vi "EVE.vi"() -> ()   [LabVIEW 2011]
uses:
  <vilib>/express/express analysis/Spectral/XNode/ExpressSpectralMeasurementsBlockNode.xnode
  <vilib>/express/express analysis/Spectral/Block/exnSpectralBlock spectral measurements RMS poly.vi
  <vilib>/picture/3D Picture Control/NI_3D Picture Control.lvlib
  <vilib>/Analysis/NI_AALPro.lvlib
  <vilib>/Analysis/2dsp.llb/Real FFT.vi
  <vilib>/Utility/file.llb/Read From Spreadsheet File (string).vi
  <vilib>/Platform/NI_3dgraph.lvlib
  <vilib>/Analysis/coordinate.llb/3D Cartesian Coordinate Rotation (Euler) (Array).vi
  <vilib>/express/express analysis/Spectral/Block/exnSpectralBlock spectral measurements RMS DDT.vi
  <vilib>/Analysis/4window.llb/Hamming Window (DBL).vi
  <vilib>/imath/engines/lvmath/Plug In/_Char/NIMS_CH_String CV to Character 2D.vi
  <vilib>/imath/engines/lvmath/Plug In/_Char/NIMS_CH_Character 2D to U8 2D.vi
  <vilib>/imath/engines/lvmath2/RunTimeEngine/ArithmeticOperatorToken/NIMS_ArithmeticOperator_multmx.vi
  <vilib>/imath/engines/lvmath2/RunTimeEngine/ArithmeticOperatorToken/NIMS_ArithmeticOperator_plus.vi
  <vilib>/imath/engines/lvmath2/RunTimeEngine/ArithmeticOperatorToken/NIMS_ArithmeticOperator_powermx(M,M).vi
  <vilib>/imathl/engines/lvmath/Functions/Error Handling/Create Error.vi
  <vilib>/imath/engines/lvmath2/RunTimeEngine/BuiltInFunctions/atan2/NIMS_atan2(A,A).vi
  <vilib>/imath/engines/lvmath2/RunTimeEngine/ErrorHandling/NIMS_Create Error From Enums.vi
  <vilib>/imath/engines/lvmath/Functions/Error Handling/MergeErrorsWrapper.vi
  <vilib>/imath/engines/lvmath2/RunTimeEngine/ArithmeticOperatorToken/NIMS_ArithmeticOperator_minus.vi
  <vilib>/imath/engines/lvmath2/RunTimeEngine/NodeEndStatement/NIMS_NodeEndStatement_Output.vi
  <vilib>/imath/engines/lvmath2/RunTimeEngine/ErrorHandling/NIMS_Finalize Error.vi
panel:
  out "Z direction  FFT 10":dbl[](graph)
  out "Z direction  FFT 9":dbl[](graph)
  out "Z direction  FFT 8":dbl[](graph)
  out "Z direction  FFT 7":dbl[](graph)
  out "Z direction  FFT 6":dbl[](graph)
  out "Z direction  FFT 5":dbl[](graph)
  in  "3D Curve":refnum<k7>(container)
  in  "Z":dbl[](array[numeric])
  in  "Y":dbl[](array[numeric])
  in  "X":dbl[](array[numeric])
  out "Z direction  FFT 4":dbl[](graph)
  out "Y direction  FFT":dbl[](graph)
  out "X direction  FFT 2":dbl[](graph)
  out "Data Selected 3":u16
  out "Data Selected 2":u16
  in  "Load in CSV File Data1":path
  in  "Tab Control 2":enum32{"Swimming", "Cycling", "Running"}(tab)
  in  "Tab Control":enum32{"Raw Accelerations", "FFT"}(tab)
  in  "Select Data to Analyse":u16(ring) items=["Data 0", "Data 1"]
  in  "Angle":sgl(knob) scale=0.0..360.0
  in  "Axis":cluster{"X":sgl, "Y":sgl, "Z":sgl}
  out "?":string[](array[string])
  out "?":string[](array[string])
  out "Data Seperated and Organised into Columns and Rows":string[][](array[string])
  out "CSV File":string[][](array[string])
  in  "Stop":bool
  out "Number of Rows in File":i32
  in  "Load in CSV File Data0":path
  in  "Translation":cluster{"X":sgl, "Y":sgl, "Z":sgl}
  out "3D Picture Control":refnum<vi>(3d-picture)
  in  "stop":bool
  in  "STL File Path":path
  in  "Reset Signal":bool
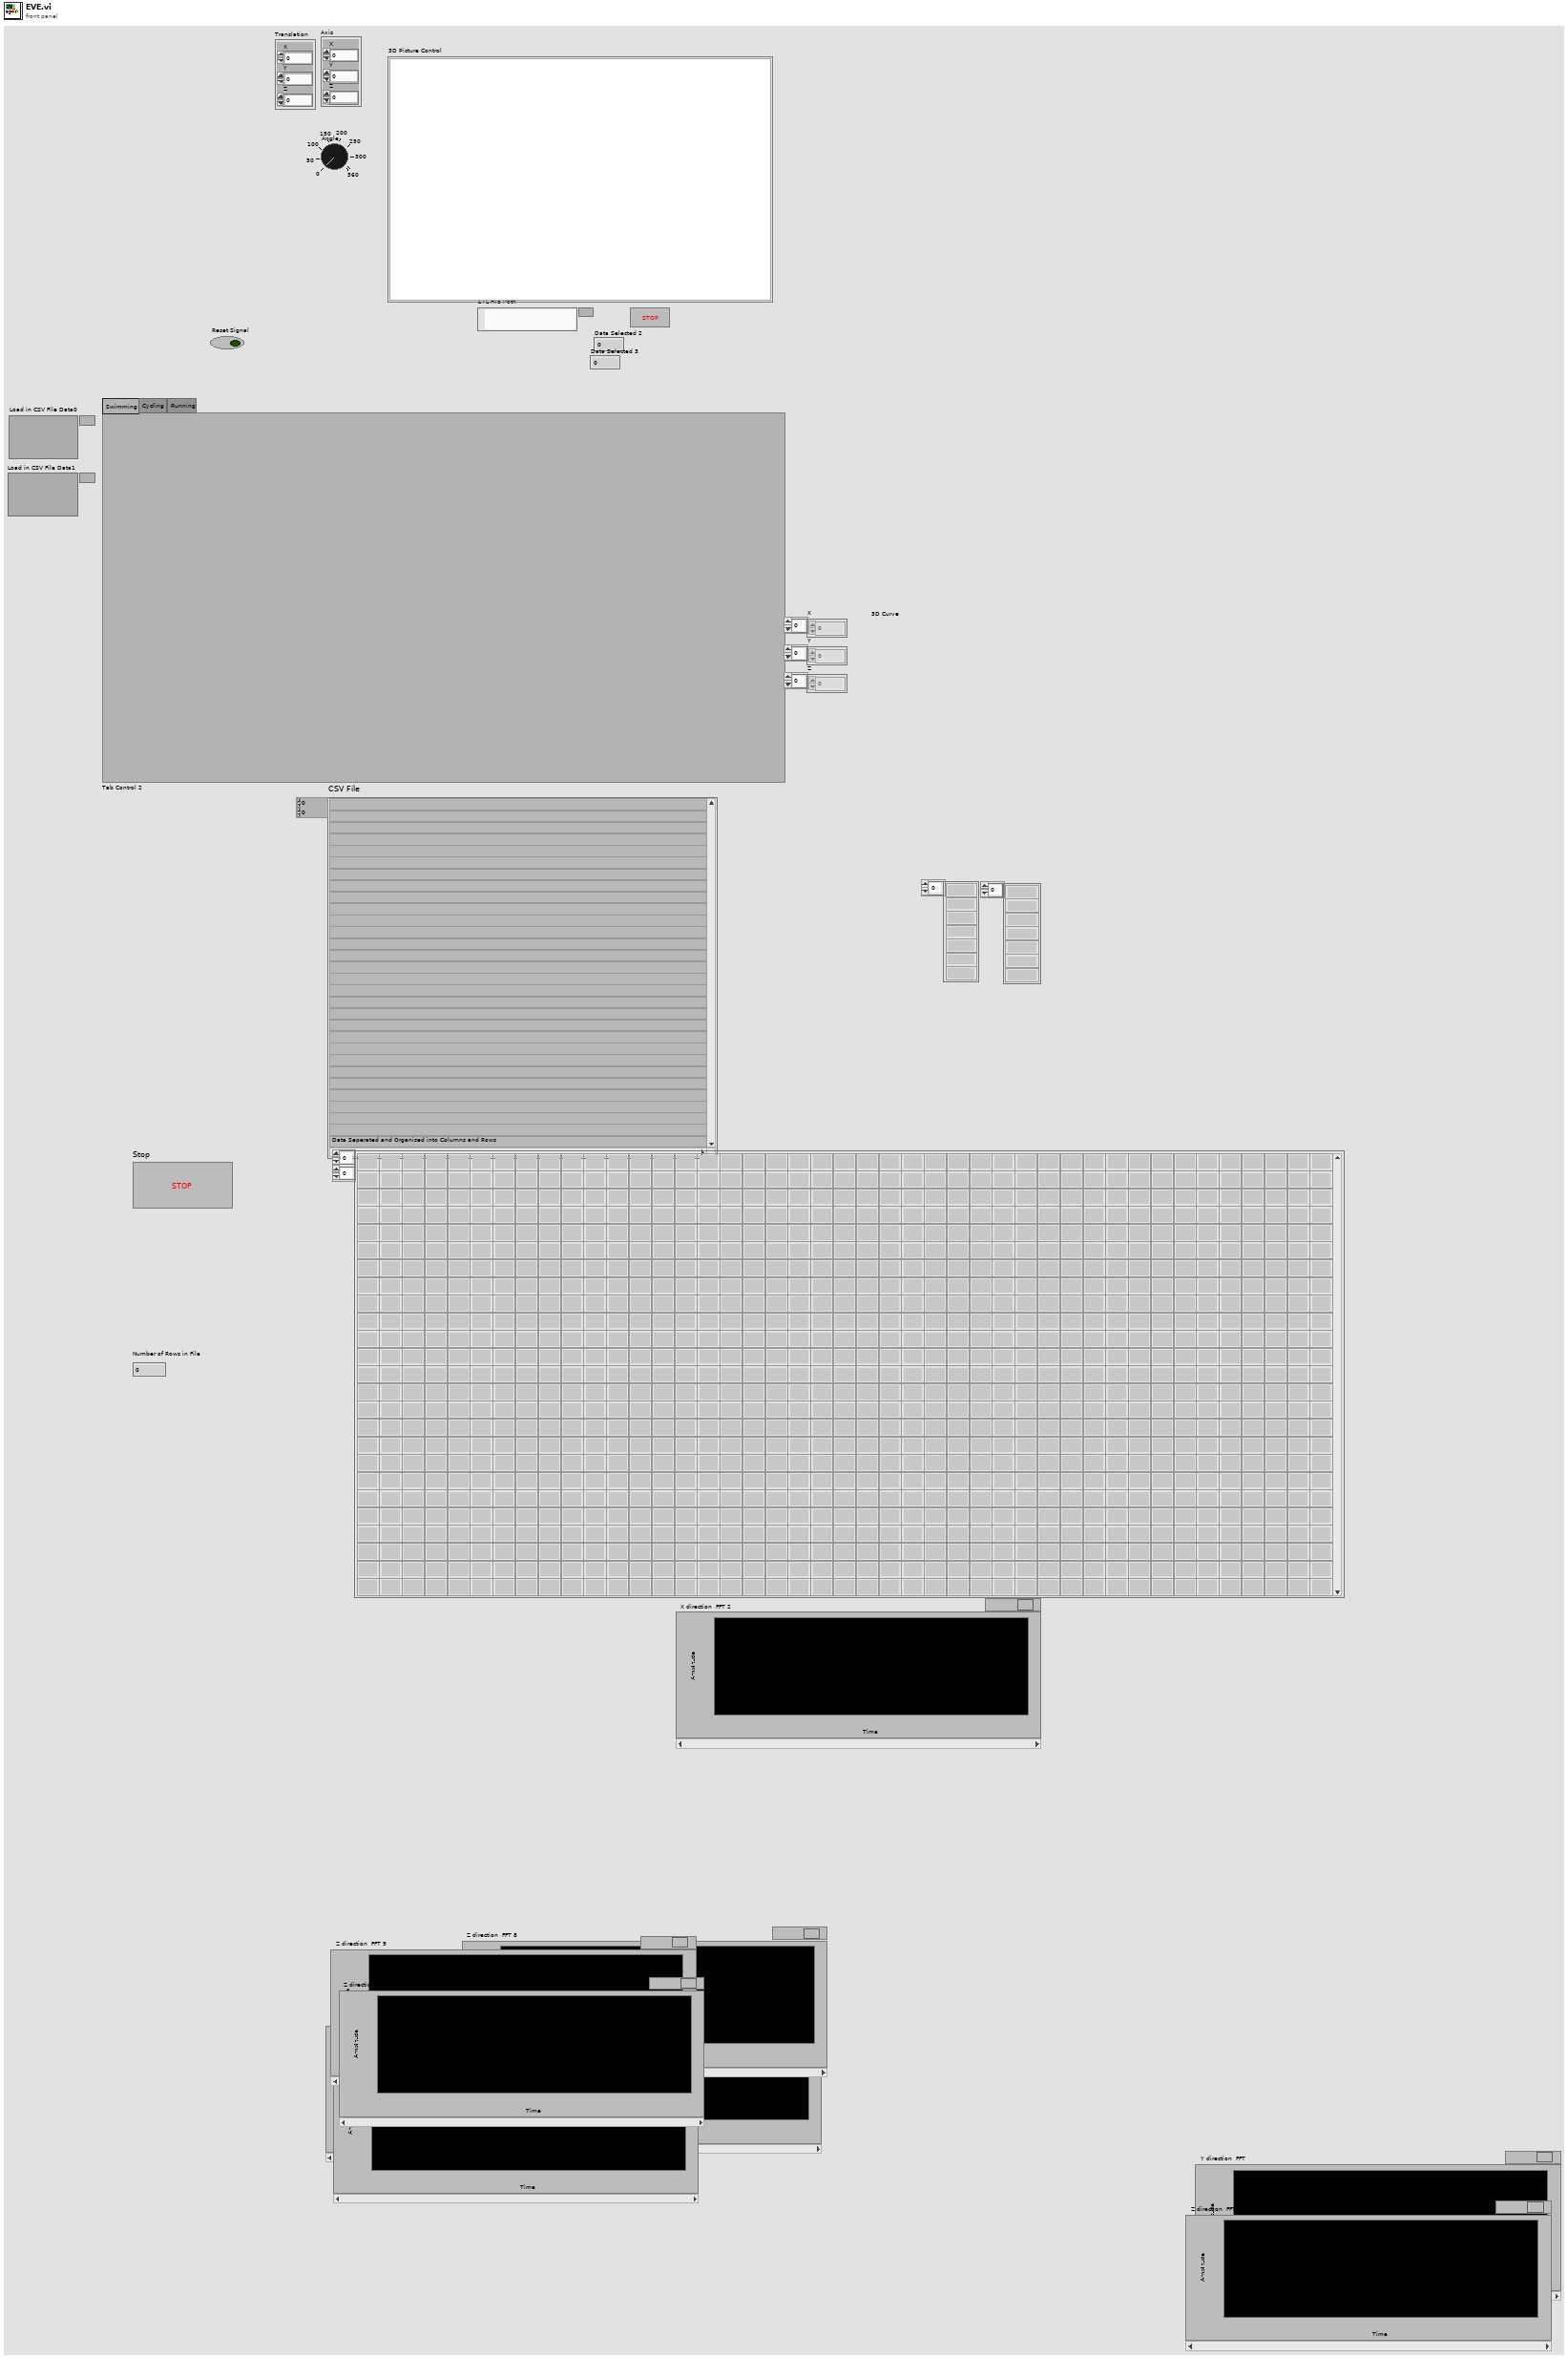
[diagram p1: front panel]
types:
  T1 = cluster{"averaging mode":u16, "weighting mode":u16, "number of averages":u32}
  T2 = cluster{"dB On (F)":bool, "unwrap phase (F)":bool, "convert to degree (F)":bool}
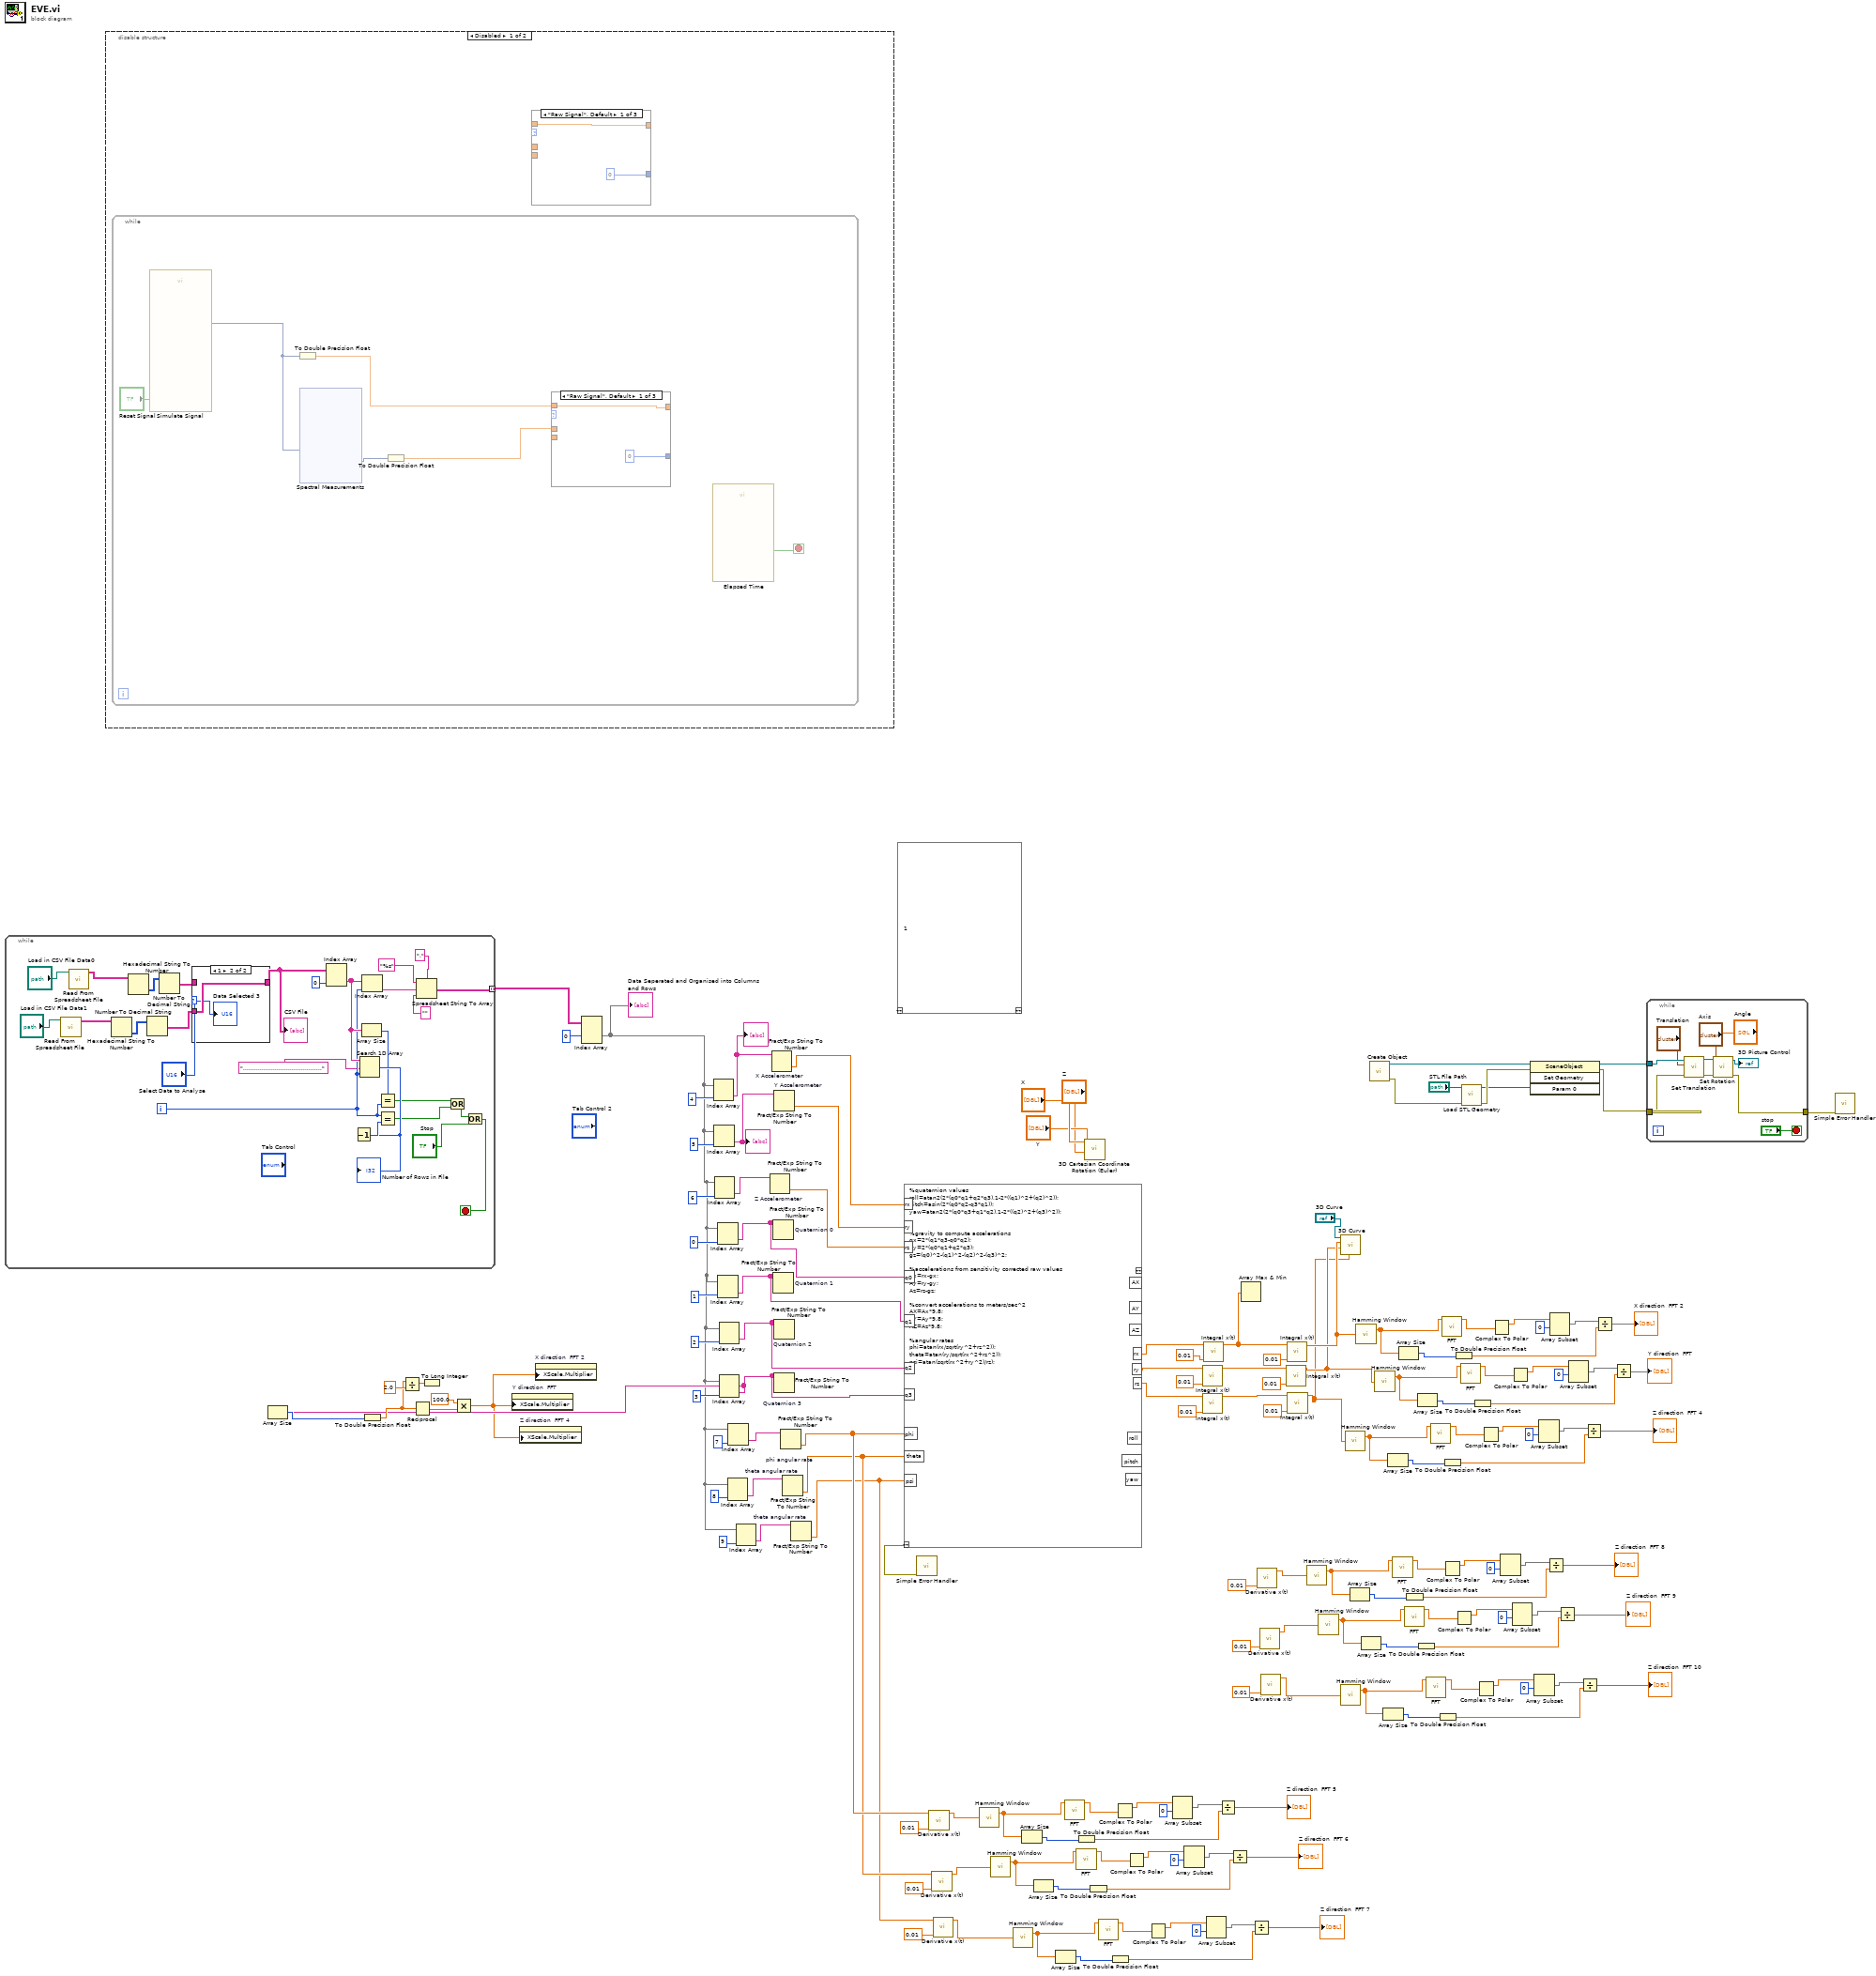
[diagram p0: block diagram]
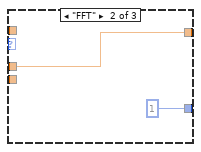
[diagram p2: hidden frame]
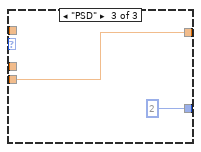
[diagram p3: hidden frame]
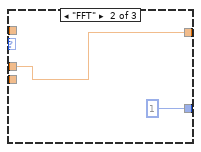
[diagram p4: hidden frame]
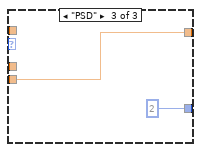
[diagram p5: hidden frame]
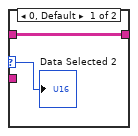
[diagram p7: hidden frame]
diagram:
  n1 = while {
    tunnel: [w173] -> w147 mode=indexing
    i -> [w168]
    stop <- w165 stop-if-true
    n2 = call-poly <vilib>:"Read From Spreadsheet File.vi"("file path (dialog if empty)"="Load in CSV File Data1") -> ("all rows"=w153:string[][])  [unwired: 6 in, 4 out]
    n3 = call-poly <vilib>:"Read From Spreadsheet File.vi"("file path (dialog if empty)"="Load in CSV File Data0") -> ("all rows"=w156:string[][])  [unwired: 6 in, 4 out]
    n4 = Hexadecimal String To Number(string=w153) -> (number=w154:u32[][])  [unwired: 2 in, 1 out]
    n5 = Hexadecimal String To Number(string=w156) -> (number=w151:u32[][])  [unwired: 2 in, 1 out]
    n6 = Number To Decimal String(number=w154) -> (decimal integer string=w155:string[][])  [unwired: 1 in]
    n7 = Number To Decimal String(number=w151) -> (decimal integer string=w152:string[][])  [unwired: 1 in]
    n8 = case shown="1" "Select Data to Analyse" {
      selector: "Select Data to Analyse" -> [w179 w180]
      tunnel: w152 -> [w178 _]
      tunnel: w155 -> [_ w181]
      tunnel: [w178 w181] -> w157
      frame 0, Default {
        "Data Selected 2" <- w179
      }
      frame 1 {
        "Data Selected 3" <- w180
      }
    }
    "CSV File" <- w157
    n9 = Index Array(array=w157, index (col)=0 ("index (row)")) -> (element=w170:string[])  [unwired: 1 in]
    n10 = Search 1D Array(1D array=w170, element=",,,,,,,,,,,,,,,,,,,,,,,,,,,,,,,,,,,,,,,,,,", start index (0)=w168) -> (index of element=w171:i32)
    "Number of Rows in File" <- w171
    n11 = Decrement(x=w171) -> (x-1=w172:i32)
    n12 = Array Size(array=w170) -> (size(s)=w169:i32)
    n13 = Index Array(array=w170, index=w168) -> (element=w159:string)
    n14 = Equal?(x=w169, y=w168) -> (x = y?=w166:bool)
    n15 = Equal?(x=w168, y=w172) -> (x = y?=w167:bool)
    n16 = Spreadsheet String To Array(delimiter (Tab)=",", format string="%s", spreadsheet string=w159, array type (2D Dbl)="" ("delimiter (Tab)")) -> (array=w173:string[][])
    n17 = Or(x=w166, y=w167) -> (x .or. y?=w163:bool)
    n18 = Or(x=w163, y="Stop") -> (x .or. y?=w165:bool)
  }
  n19 = disable-structure shown="Disabled" {
    frame Disabled {
      n20 = while {
        stop <- w190 stop-if-true
        n21 = call "Simulate Signal"("Reset Signal"="Reset Signal") -> ("Sine"=w193:dynamicdata, "Frequency"=w194:dbl)  [unwired: 12 in, 1 out]
        n22 = To Double Precision Float(number=w193) -> (double precision float=w192:dbl)
        n23 = xnode "Spectral Measurements"("Signals"=w193) -> ("FFT - (RMS)"=w196:dynamicdata)  [unwired: 1 in, 2 out]
        n24 = To Double Precision Float(number=w196) -> (double precision float=w191:dbl)
        n25 = case shown="\"Raw Signal\", Default" w189 {
          tunnel: w192 -> [w197 _ _]
          tunnel: w191 -> [_ w199 _]
          tunnel: _ -> [_ _ w201]
          tunnel: [0 1 2] -> _
          tunnel: [w197 w199 w201] -> w188
          frame "Raw Signal", Default {
          }
          frame "FFT" {
          }
          frame "PSD" {
          }
        }
        n26 = call "Elapsed Time"() -> ("Time has Elapsed"=w190:bool)  [unwired: 12 in, 7 out]
      }
      n27 = case shown="Default, \"Data 1\"" {
        selector: _ -> [_ _ _]
        tunnel: _ -> [w182 _ _]
        tunnel: _ -> [_ w184 _]
        tunnel: _ -> [_ _ w186]
        tunnel: [0 1 2] -> _
        tunnel: [w182 w184 w186] -> _
        frame "Raw Signal", Default {
        }
        frame "FFT" {
        }
        frame "PSD" {
        }
      }
    }
    frame Enabled {
    }
  }
  n28 = Index Array(array=w147, index (dim 1)=0 ("index (page)")) -> (element=w66:string[][])  [unwired: 2 in]
  "Data Seperated and Organised into Columns and Rows" <- w66
  n29 = Index Array(array=w66, index (col)=4 ("disabled index (col)")) -> (element=w149:string[])  [unwired: 1 in]
  "?" <- w149
  n30 = Index Array(array=w66, index (col)=5 ("disabled index (col)")) -> (element=w148:string[])  [unwired: 1 in]
  "?" <- w148
  n31 = Index Array(array=w66, index (col)=6 ("disabled index (col)")) -> (element=w143:string[])  [unwired: 1 in]
  n32 = Index Array(array=w66, index (col)=0 ("disabled index (col)")) -> (element=w137:string[])  [unwired: 1 in]
  n33 = Index Array(array=w66, index (col)=1 ("disabled index (col)")) -> (element=w136:string[])  [unwired: 1 in]
  n34 = Index Array(array=w66, index (col)=2 ("disabled index (col)")) -> (element=w135:string[])  [unwired: 1 in]
  n35 = Index Array(array=w66, index (col)=3 ("disabled index (col)")) -> (element=w100:string[])  [unwired: 1 in]
  n36 = Array Size(array=w100) -> (size(s)=w101:i32)
  n37 = To Double Precision Float(number=w101) -> (double precision float=w106:dbl)
  n38 = Divide(x=w106, y=2.0) -> (x/y=w104:dbl)
  n39 = Reciprocal(x=w106) -> (1/x=w105:dbl)
  n40 = To Long Integer(number=w104) -> ()  [unwired: 1 out]
  n41 = Multiply(x=100.0 ("double precision float"), y=w105) -> (x*y=w97:dbl)
  n42 = property on="Y direction  FFT" class="WFChart (strict)"("XScale.Multiplier"=w97) -> ()  [unwired: 2 in, 2 out]
  n43 = property on="Z direction  FFT 4" class="WFChart (strict)"("XScale.Multiplier"=w97) -> ()  [unwired: 2 in, 2 out]
  n44 = property on="X direction  FFT 2" class="WFChart (strict)"("XScale.Multiplier"=w97) -> ()  [unwired: 2 in, 2 out]
  n45 = Index Array(array=w66, index (col)=8 ("disabled index (col)")) -> (element=w69:string[])  [unwired: 1 in]
  n46 = Index Array(array=w66, index (col)=7 ("disabled index (col)")) -> (element=w71:string[])  [unwired: 1 in]
  n47 = Index Array(array=w66, index (col)=9 ("disabled index (col)")) -> (element=w67:string[])  [unwired: 1 in]
  n48 = Fract/Exp String To Number "Z Accelerometer"(string=w143) -> (number=w138:dbl[])  [unwired: 3 in, 1 out]
  n49 = Fract/Exp String To Number "X Accelerometer"(string=w149) -> (number=w132:dbl[])  [unwired: 3 in, 1 out]
  n50 = Fract/Exp String To Number "Quaternion 0"(string=w137) -> ()  [unwired: 3 in, 2 out]
  n51 = Fract/Exp String To Number "Quaternion 1"(string=w136) -> ()  [unwired: 3 in, 2 out]
  n52 = Fract/Exp String To Number "Y Accelerometer"(string=w148) -> (number=w133:dbl[])  [unwired: 3 in, 1 out]
  n53 = Fract/Exp String To Number "Quaternion 2"(string=w135) -> ()  [unwired: 3 in, 2 out]
  n54 = Fract/Exp String To Number "Quaternion 3"(string=w100) -> ()  [unwired: 3 in, 2 out]
  n55 = Fract/Exp String To Number "phi angular rate"(string=w71) -> (number=w65:dbl[])  [unwired: 3 in, 1 out]
  n56 = Fract/Exp String To Number "theta angular rate"(string=w69) -> (number=w61:dbl[])  [unwired: 3 in, 1 out]
  n57 = Fract/Exp String To Number "theta angular rate"(string=w67) -> (number=w60:dbl[])  [unwired: 3 in, 1 out]
  n58 = mathscript code="1"() -> ()  [unwired: 1 in, 1 out]
  n59 = call <vilib>:"Simple Error Handler.vi"() -> ("error out"=w134:errorcluster)  [unwired: 2 in, 7 out]
  n60 = mathscript code="%quaternion values\nroll=atan2(2*(q0*q1+q2*q3),1-2*((q1)^2+(q2)^2));\npitch=asin(2*(q0*q2-q3*q1));\nyaw=atan2(2*(q0*q3+q1*q2),1-2*((q2)^2+(q3)^2));\n\n\n%gravity to compute accelerations\ngx=2*(q1*q3-q0*q2);\ngy=2*(q0*q1+q2*q3);\ngz=(q0)^2-(q1)^2-(q2)^2-(q3)^2;\n\n%accelerations from sensitivity corrected raw values\nAx=rx-gx;\nAy=ry-gy;\nAz=rz-gz;\n\n%convert accelerations to meters/sec^2\nAX=Ax*9.8;\nAY=Ay*9.8;\nAZ=Az*9.8;\n\n%angular rates\nphi=atan(rx/sqrt(ry^2+rz^2));\ntheta=atan(ry/sqrt(rx^2+rz^2));\npsi=atan(sqrt(rx^2+ry^2)/rz);"("??"=w134, "q0"=w137, "q1"=w136, "q2"=w135, "q3"=w100, "rz"=w138, "ry"=w133, "rx"=w132, "phi"=w65, "theta"=w61, "psi"=w60) -> ("rx"=w131:dbl[], "ry"=w129:dbl[], "rz"=w127:dbl[])  [unwired: 7 out]
  n61 = call <vilib>:"Derivative x(t).vi"("dt"=0.01, "X"=w65) -> ("dX/dt"=w51:dbl[])  [unwired: 8 in, 1 out]
  n62 = call <vilib>:"Derivative x(t).vi"("dt"=0.01, "X"=w61) -> ("dX/dt"=w42:dbl[])  [unwired: 8 in, 1 out]
  n63 = call <vilib>:"Derivative x(t).vi"("dt"=0.01, "X"=w60) -> ("dX/dt"=w33:dbl[])  [unwired: 8 in, 1 out]
  n64 = call-poly <vilib>:"Hamming Window.vi"("X"=w51) -> ("Windowed X"=w53:dbl[])  [unwired: 1 out]
  n65 = call-poly <vilib>:"Hamming Window.vi"("X"=w42) -> ("Windowed X"=w44:dbl[])  [unwired: 1 out]
  n66 = call-poly <vilib>:"Hamming Window.vi"("X"=w33) -> ("Windowed X"=w35:dbl[])  [unwired: 1 out]
  n67 = Array Size(array=w53) -> (size(s)=w56:i32)
  n68 = Array Size(array=w44) -> (size(s)=w47:i32)
  n69 = Array Size(array=w35) -> (size(s)=w38:i32)
  n70 = call-poly <vilib>:"FFT.vi"("X"=w53) -> ("FFT {X}"=w59:cdb[])  [unwired: 9 in, 1 out]
  n71 = call-poly <vilib>:"FFT.vi"("X"=w44) -> ("FFT {X}"=w50:cdb[])  [unwired: 9 in, 1 out]
  n72 = To Double Precision Float(number=w56) -> (double precision float=w54:dbl)
  n73 = call-poly <vilib>:"3D Cartesian Coordinate Rotation (Euler).vi"("Z"="Z", "Y"="Y", "X"="X") -> ()  [unwired: 5 in, 4 out]
  n74 = To Double Precision Float(number=w47) -> (double precision float=w45:dbl)
  n75 = call-poly <vilib>:"FFT.vi"("X"=w35) -> ("FFT {X}"=w41:cdb[])  [unwired: 9 in, 1 out]
  n76 = To Double Precision Float(number=w38) -> (double precision float=w36:dbl)
  n77 = Complex To Polar(r * e^(i*theta)=w59) -> (r=w58:dbl[])  [unwired: 1 out]
  n78 = Complex To Polar(r * e^(i*theta)=w50) -> (r=w49:dbl[])  [unwired: 1 out]
  n79 = Complex To Polar(r * e^(i*theta)=w41) -> (r=w40:dbl[])  [unwired: 1 out]
  n80 = Array Subset(array=w58, index=0) -> (w55:dbl[])  [unwired: 1 in]
  n81 = Array Subset(array=w49, index=0) -> (w46:dbl[])  [unwired: 1 in]
  n82 = call <vilib>:"Integral x(t).vi"("dt"=0.01, "X"=w129) -> ("Integral X"=w130:dbl[])  [unwired: 8 in, 1 out]
  n83 = call <vilib>:"Integral x(t).vi"("dt"=0.01, "X"=w127) -> ("Integral X"=w128:dbl[])  [unwired: 8 in, 1 out]
  n84 = call <vilib>:"Integral x(t).vi"("dt"=0.01, "X"=w131) -> ("Integral X"=w76:dbl[])  [unwired: 8 in, 1 out]
  n85 = Array Subset(array=w40, index=0) -> (w37:dbl[])  [unwired: 1 in]
  n86 = Divide(x=w55, y=w54) -> (x/y=→"Z direction  FFT 5":dbl[])
  n87 = Divide(x=w46, y=w45) -> (x/y=→"Z direction  FFT 6":dbl[])
  n88 = Array Max & Min(array=w76) -> ()  [unwired: 4 out]
  n89 = Divide(x=w37, y=w36) -> (x/y=→"Z direction  FFT 7":dbl[])
  n90 = call <vilib>:"Derivative x(t).vi"("dt"=0.01) -> ("dX/dt"=w19:dbl[])  [unwired: 9 in, 1 out]
  n91 = call <vilib>:"Derivative x(t).vi"("dt"=0.01) -> ("dX/dt"=w10:dbl[], "X"=w29:dbl[])  [unwired: 8 in, 1 out]
  n92 = call <vilib>:"Derivative x(t).vi"("dt"=0.01) -> ("dX/dt"=w1:dbl[], "X"=w28:dbl[])  [unwired: 8 in, 1 out]
  n93 = call <vilib>:"Integral x(t).vi"("dt"=0.01, "X"=w130) -> ("Integral X"=w89:dbl[])  [unwired: 8 in, 1 out]
  n94 = call <vilib>:"Integral x(t).vi"("dt"=0.01, "X"=w76) -> ("Integral X"=w102:dbl[])  [unwired: 8 in, 1 out]
  n95 = call <vilib>:"Integral x(t).vi"("dt"=0.01, "X"=w128) -> ("Integral X"=w80:dbl[])  [unwired: 8 in, 1 out]
  n96 = call-poly <vilib>:"Hamming Window.vi"("X"=w19) -> ("Windowed X"=w21:dbl[])  [unwired: 1 out]
  n97 = call-poly <vilib>:"Hamming Window.vi"("X"=w10) -> ("Windowed X"=w12:dbl[])  [unwired: 1 out]
  n98 = call <vilib>:"3D Curve.vi"("z vector"=w80, "y vector"=w89, "x vector"=w102, "3D graph"="3D Curve") -> ()  [unwired: 6 in, 2 out]
  n99 = call-poly <vilib>:"Hamming Window.vi"("X"=w1) -> ("Windowed X"=w3:dbl[])  [unwired: 1 out]
  n100 = call-poly <vilib>:"Hamming Window.vi"("X"=w80) -> ("Windowed X"=w81:dbl[])  [unwired: 1 out]
  n101 = Array Size(array=w21) -> (size(s)=w24:i32)
  n102 = call-poly <vilib>:"Hamming Window.vi"("X"=w102) -> ("Windowed X"=w108:dbl[])  [unwired: 1 out]
  n103 = Array Size(array=w12) -> (size(s)=w15:i32)
  n104 = call <vilib>:"Create Object.vi"() -> ("error out"=w125:errorcluster, "Scene:New Object"=w124:refnum<vi>)  [unwired: 2 in, 8 out]
  n105 = call-poly <vilib>:"Hamming Window.vi"("X"=w89) -> ("Windowed X"=w90:dbl[])  [unwired: 1 out]
  n106 = Array Size(array=w3) -> (size(s)=w6:i32)
  n107 = Array Size(array=w81) -> (size(s)=w84:i32)
  n108 = call-poly <vilib>:"FFT.vi"("X"=w21) -> ("FFT {X}"=w27:cdb[])  [unwired: 9 in, 1 out]
  n109 = Array Size(array=w108) -> (size(s)=w111:i32)
  n110 = call-poly <vilib>:"FFT.vi"("X"=w12) -> ("FFT {X}"=w18:cdb[])  [unwired: 9 in, 1 out]
  n111 = To Double Precision Float(number=w24) -> (double precision float=w22:dbl)
  n112 = To Double Precision Float(number=w15) -> (double precision float=w13:dbl)
  n113 = Array Size(array=w90) -> (size(s)=w93:i32)
  n114 = call-poly <vilib>:"FFT.vi"("X"=w3) -> ("FFT {X}"=w9:cdb[])  [unwired: 9 in, 1 out]
  n115 = call-poly <vilib>:"FFT.vi"("X"=w81) -> ("FFT {X}"=w87:cdb[])  [unwired: 9 in, 1 out]
  n116 = To Double Precision Float(number=w6) -> (double precision float=w4:dbl)
  n117 = call-poly <vilib>:"FFT.vi"("X"=w108) -> ("FFT {X}"=w114:cdb[])  [unwired: 9 in, 1 out]
  n118 = To Double Precision Float(number=w84) -> (double precision float=w82:dbl)
  n119 = Complex To Polar(r * e^(i*theta)=w27) -> (r=w26:dbl[])  [unwired: 1 out]
  n120 = To Double Precision Float(number=w111) -> (double precision float=w109:dbl)
  n121 = Complex To Polar(r * e^(i*theta)=w18) -> (r=w17:dbl[])  [unwired: 1 out]
  n122 = call-poly <vilib>:"FFT.vi"("X"=w90) -> ("FFT {X}"=w96:cdb[])  [unwired: 9 in, 1 out]
  n123 = call <vilib>:"Load STL Geometry.vi"("error in (no error)"=w125, "Model File"="STL File Path") -> ("error out"=w123:errorcluster, "New Mesh Refnum"=w116:refnum<vi>)  [unwired: 8 out]
  n124 = To Double Precision Float(number=w93) -> (double precision float=w91:dbl)
  n125 = Complex To Polar(r * e^(i*theta)=w9) -> (r=w8:dbl[])  [unwired: 1 out]
  n126 = Complex To Polar(r * e^(i*theta)=w87) -> (r=w86:dbl[])  [unwired: 1 out]
  n127 = Complex To Polar(r * e^(i*theta)=w114) -> (r=w113:dbl[])  [unwired: 1 out]
  n128 = Array Subset(array=w26, index=0) -> (w23:dbl[])  [unwired: 1 in]
  n129 = Complex To Polar(r * e^(i*theta)=w96) -> (r=w95:dbl[])  [unwired: 1 out]
  n130 = Array Subset(array=w17, index=0) -> (w14:dbl[])  [unwired: 1 in]
  n131 = invoke class="SceneObject" method="Set Geometry"(reference=w124, error in=w123, "Param 0"=w116) -> (reference out=w120:refnum<vi>, error out=w122:errorcluster)  [unwired: 1 in, 2 out]
  n132 = Array Subset(array=w8, index=0) -> (w5:dbl[])  [unwired: 1 in]
  n133 = Array Subset(array=w86, index=0) -> (w83:dbl[])  [unwired: 1 in]
  n134 = Divide(x=w23, y=w22) -> (x/y=→"Z direction  FFT 8":dbl[])
  n135 = Array Subset(array=w113, index=0) -> (w110:dbl[])  [unwired: 1 in]
  n136 = Divide(x=w14, y=w13) -> (x/y=→"Z direction  FFT 9":dbl[])
  n137 = Array Subset(array=w95, index=0) -> (w92:dbl[])  [unwired: 1 in]
  n138 = Divide(x=w5, y=w4) -> (x/y=→"Z direction  FFT 10":dbl[])
  n139 = Divide(x=w83, y=w82) -> (x/y=→"Z direction  FFT 4":dbl[])
  n140 = Divide(x=w110, y=w109) -> (x/y=→"X direction  FFT 2":dbl[])
  n141 = Divide(x=w92, y=w91) -> (x/y=→"Y direction  FFT":dbl[])
  n142 = while {
    tunnel: w120 -> [w221]
    tunnel: w122 -> [w220]
    tunnel: [w215] -> w121
    stop <- "stop" stop-if-true
    n143 = call <vilib>:"Set Translation.vi"("error in (no error)"=w220, "Translation"="Translation", "Scene Object"=w221) -> ("error out"=w218:errorcluster, "Translated Object"=w217:refnum<vi>)  [unwired: 7 in]
    n144 = call <vilib>:"Set Rotation.vi"("error in (no error)"=w218, "Angle"="Angle", "Axis"="Axis", "Scene Object"=w217) -> ("error out"=w215:errorcluster, "Rotated Scene Object"=→"3D Picture Control":refnum<vi>)  [unwired: 6 in]
  }
  n145 = call <vilib>:"Simple Error Handler.vi"("error in (no error)"=w121) -> ()  [unwired: 1 in, 8 out]
